vi "WriteGlobalVariables.vi"() -> ()   [LabVIEW 2014]
uses:
  GlobalVariables.vi
panel:
  in  "stop":bool
  in  "Time in Mins.":i32=15
  in  "Write to File Path":path
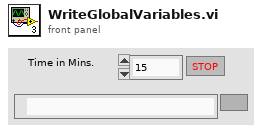
[diagram p1: front panel]
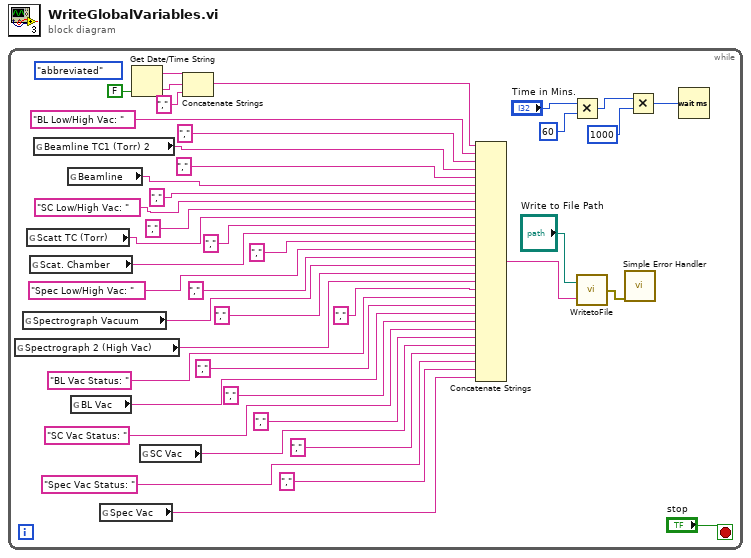
[diagram p0: block diagram]
diagram:
  n1 = while {
    stop <- "stop" stop-if-true
    (unwired) enum16{"short", "long", "abbreviated"}."abbreviated" ("date format (0)")
    n2 = global read "GlobalVariables.vi" "Spectrograph 2 (High Vac)"() -> (w20:string)
    n3 = global read "GlobalVariables.vi" "Spectrograph Vacuum"() -> (w22:string)
    n4 = global read "GlobalVariables.vi" "Scatt TC (Torr)"() -> (w28:string)
    n5 = global read "GlobalVariables.vi" "Scat. Chamber"() -> (w26:string)
    n6 = global read "GlobalVariables.vi" "Beamline TC1 (Torr) 2"() -> (w34:string)
    n7 = global read "GlobalVariables.vi" "Beamline"() -> (w32:string)
    n8 = global read "GlobalVariables.vi" "BL Vac"() -> (w16:string)
    n9 = global read "GlobalVariables.vi" "Spec Vac"() -> (w8:string)
    n10 = Get Date/Time String(want seconds? (F)=FALSE) -> (date string=w42:string, time string=w41:string)  [unwired: 2 in]
    n11 = global read "GlobalVariables.vi" "SC Vac"() -> (w12:string)
    n12 = Concatenate Strings(w42, w41, "," ("string")) -> (w40:string)
    n13 = Concatenate Strings(w40, "BL Low/High Vac: " ("string"), "," ("string"), w34, "," ("string"), w32, "," ("string"), "SC Low/High Vac: " ("string"), "," ("string"), w28, "," ("string"), w26, "," ("string"), "Spec Low/High Vac: " ("string"), "," ("string"), w22, "," ("string"), w20, "," ("string"), "BL Vac Status: " ("string"), "," ("string"), w16, "," ("string"), "SC Vac Status: " ("string"), "," ("string"), w12, "," ("string"), "Spec Vac Status: " ("string"), "," ("string"), w8) -> (w37:string)
    n14 = Multiply(x="Time in Mins.", y=60) -> (x*y=w5:i32)
    n15 = call "WritetoFile.vi"("text"=w37, "Path"="Write to File Path") -> ("error out"=w38:errorcluster)
    n16 = call <vilib>:"Simple Error Handler.vi"("error in (no error)"=w38) -> ()  [unwired: 4 in, 5 out]
    n17 = Multiply(x=w5, y=1000) -> (x*y=w3:i32)
    n18 = Wait (ms)(milliseconds to wait=w3) -> ()  [unwired: 1 out]
  }
